vi "Read Unit label.vi"(9 "GraphScale in":refnum<class "GraphScale.lvclass">) -> (3 "GraphScale out":refnum<class "GraphScale.lvclass">, 4 "Unit label":refnum<class "Text.lvclass">)   [LabVIEW 2014, in "Raspberry Pi Compatible Compiler for LabVIEW.lvlib" / "GraphScale.lvclass"]
uses:
  GraphScale.lvclass
  Text/Text.lvclass
  GraphScale.lvclass/GraphScale.ctl
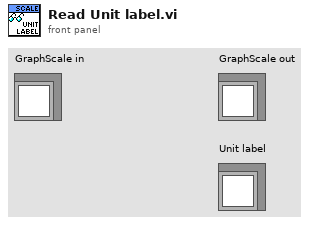
[diagram p1: front panel]
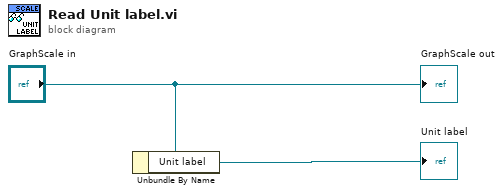
[diagram p0: block diagram]
diagram:
  n1 = Unbundle By Name("GraphScale in") -> ("Unit label"=→"Unit label":refnum<class "Text.lvclass">)
  "GraphScale out" <- "GraphScale in"
